vi "GSTOP INIT.vi"(7 "error in (no error)":errorcluster) -> (8 "error out":errorcluster)   [LabVIEW 2017, in "GSTOP.lvlib"]
doc: "Initializes the STOP FGV. If an incoming error cluster is in error state, the global stop flag is immediately set to TRUE.\n------\n初始化 STOP FGV；若输入错误簇为错误状态，则立即将全局停止位置为 TRUE。"
uses:
  GSTOP.lvlib
  _def_oper.ctl
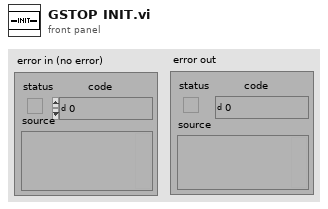
[diagram p1: front panel]
types:
  T1 = typedef "GSTOP.lvlib/_def_oper.ctl" = enum16{"init", "reset", "get", "set"}
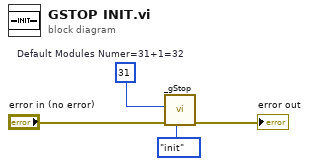
[diagram p0: block diagram]
diagram:
  w1 = u32 31  # Default Modules Numer=31+1=32
  n1 = call "_gStop.vi"("op"=_def_oper."init", "error in (no error)"="error in (no error)", "index(-1 for All)"=w1) -> ("error out"=→"error out":errorcluster)  [unwired: 7 in, 1 out]
